vi "isLeapYear (integer).vi"(2 "Year (0: this year)":i32) -> (7 "is Leap Year?":bool)   [LabVIEW 2017]
doc: "Evaluates if the year is a leap year (366 days)"
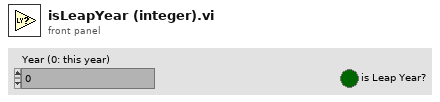
[diagram p1: front panel]
types:
  T1 = typedef "LVDateTimeRec.ctl" = cluster{"fractional second":dbl, "second":i32, "minute":i32, "hour":i32, "day of month":i32, "month":i32, "year":i32, "day of week":i32, "day of year":i32, "DST":i32}
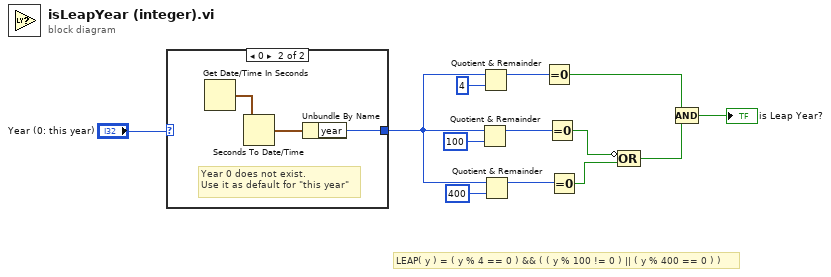
[diagram p0: block diagram]
diagram:
  # "LEAP( y ) = ( y % 4 == 0 ) && ( ( y % 100 != 0 ) || ( y % 400 == 0 ) )"
  n1 = case shown="0" "Year (0: this year)" {
    selector: "Year (0: this year)" -> [w14 _]
    tunnel: [w14 w15] -> w1
    frame Default {
    }
    frame 0 {
      # "Year 0 does not exist.\nUse it as default for \"this year\""
      n2 = Get Date/Time In Seconds() -> (seconds since 1Jan1904=w17:timestamp)
      n3 = Seconds To Date/Time(time stamp (now)=w17) -> (date time rec=w16:T1)  [unwired: 1 in]
      n4 = Unbundle By Name(w16) -> ("year"=w15:i32)
    }
  }
  n5 = Quotient & Remainder(x=w1, y=100) -> (x-y*floor(x/y)=w6:i32)  [unwired: 1 out]
  n6 = Quotient & Remainder(x=w1, y=4) -> (x-y*floor(x/y)=w10:i32)  [unwired: 1 out]
  n7 = Quotient & Remainder(x=w1, y=400) -> (x-y*floor(x/y)=w4:i32)  [unwired: 1 out]
  n8 = Equal To 0?(x=w10) -> (x = 0?=w9:bool)
  n9 = Equal To 0?(x=w6) -> (x = 0?=w5:bool)
  n10 = Equal To 0?(x=w4) -> (x = 0?=w3:bool)
  n11 = Compound Arithmetic op=OR(invert w5, w3) -> (w7:bool)
  n12 = Compound Arithmetic op=AND(w9, w7) -> (→"is Leap Year?":bool)
